vi "Test - Tagging.vi"   [LabVIEW 2023]
doc: "This VI serves as the target VI for the Tagging.vi example. Do not save changes to this VI."
panel:
  # "DO NOT SAVE CHANGES TO THIS VI. Changing this VI might prevent the Tagging.vi example from demonstrating its scripting task."
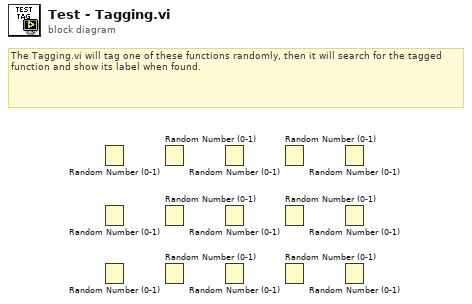
[diagram p0: block diagram]
diagram:
  # "The Tagging.vi will tag one of these functions randomly, then it will search for the tagged function and show its label when found."
  n1 = Random Number (0-1)() -> ()  [unwired: 1 out]
  n2 = Random Number (0-1)() -> ()  [unwired: 1 out]
  n3 = Random Number (0-1)() -> ()  [unwired: 1 out]
  n4 = Random Number (0-1)() -> ()  [unwired: 1 out]
  n5 = Random Number (0-1)() -> ()  [unwired: 1 out]
  n6 = Random Number (0-1)() -> ()  [unwired: 1 out]
  n7 = Random Number (0-1)() -> ()  [unwired: 1 out]
  n8 = Random Number (0-1)() -> ()  [unwired: 1 out]
  n9 = Random Number (0-1)() -> ()  [unwired: 1 out]
  n10 = Random Number (0-1)() -> ()  [unwired: 1 out]
  n11 = Random Number (0-1)() -> ()  [unwired: 1 out]
  n12 = Random Number (0-1)() -> ()  [unwired: 1 out]
  n13 = Random Number (0-1)() -> ()  [unwired: 1 out]
  n14 = Random Number (0-1)() -> ()  [unwired: 1 out]
  n15 = Random Number (0-1)() -> ()  [unwired: 1 out]
